vi "Lab4(III).vi"() -> ()   [LabVIEW 2021]
panel:
  out "7":bool
  out "6":bool
  out "3":bool
  out "5":bool
  out "4":bool
  out "2":bool
  out "1":bool
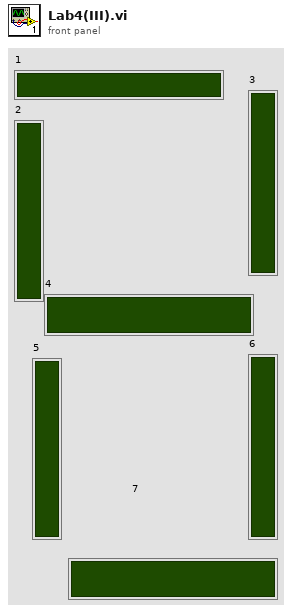
[diagram p1: front panel]
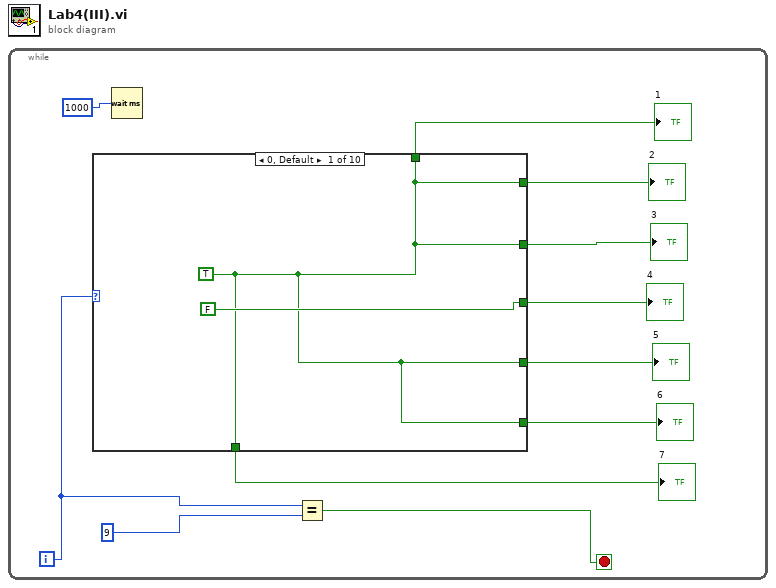
[diagram p0: block diagram]
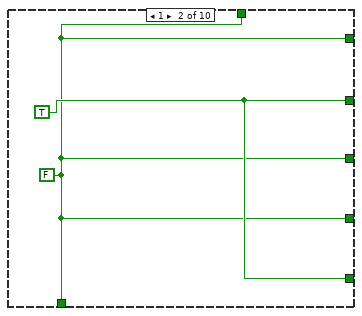
[diagram p2: hidden frame]
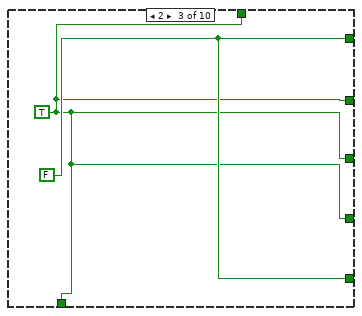
[diagram p3: hidden frame]
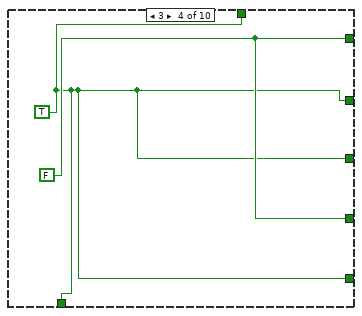
[diagram p4: hidden frame]
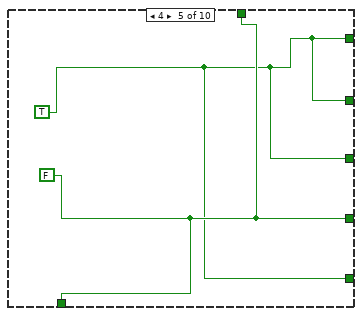
[diagram p5: hidden frame]
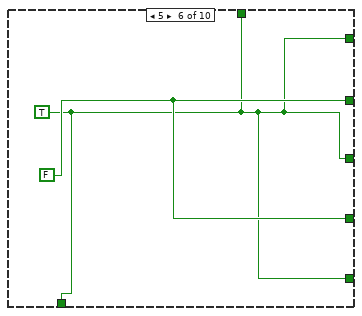
[diagram p6: hidden frame]
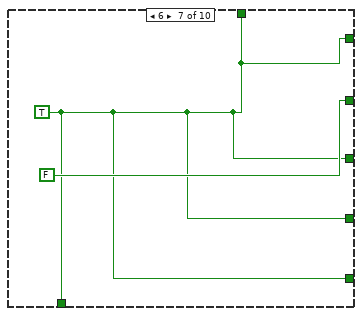
[diagram p7: hidden frame]
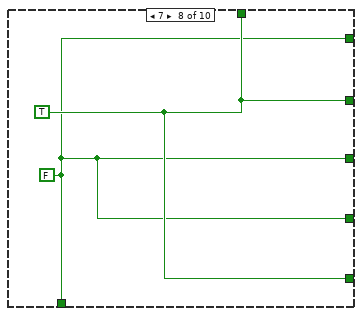
[diagram p8: hidden frame]
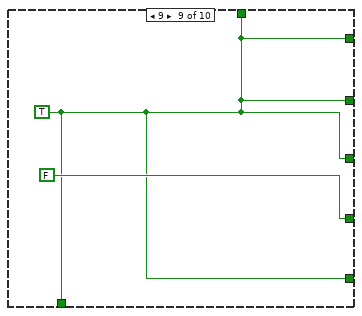
[diagram p9: hidden frame]
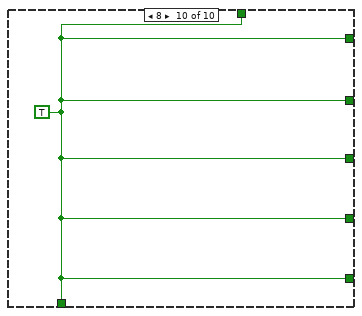
[diagram p10: hidden frame]
diagram:
  n1 = while {
    i -> [w10]
    stop <- w9 stop-if-true
    n2 = case shown="0, Default" w10 {
      tunnel: [w12 w14 w16 w18 w21 w22 w24 w27 w28 w30] -> w8
      tunnel: [w12 w15 w16 w18 w20 w23 FALSE w27 w28 w30] -> w7
      tunnel: [w12 w15 w17 w18 w20 w22 w24 w27 w28 w30] -> w6
      tunnel: [w12 w14 w17 w19 w20 w22 w24 w26 w28 w30] -> w5
      tunnel: [FALSE w14 w16 w18 w20 w22 w24 w26 w28 w30] -> w4
      tunnel: [w12 w14 w16 w19 w21 w23 w24 w26 FALSE w30] -> w3
      tunnel: [w12 w14 w16 w18 w21 w22 w24 w26 w28 w30] -> w2
      frame 0, Default {
        w12 = TRUE
      }
      frame 1 {
        w15 = TRUE
        w14 = FALSE
      }
      frame 2 {
        w16 = TRUE
        w17 = FALSE
      }
      frame 3 {
        w18 = TRUE
        w19 = FALSE
      }
      frame 4 {
        w20 = TRUE
        w21 = FALSE
      }
      frame 5 {
        w22 = TRUE
        w23 = FALSE
      }
      frame 6 {
        w24 = TRUE
      }
      frame 7 {
        w27 = TRUE
        w26 = FALSE
      }
      frame 9 {
        w28 = TRUE
      }
      frame 8 {
        w30 = TRUE
      }
    }
    "1" <- w8
    "2" <- w5
    "4" <- w4
    "5" <- w3
    "3" <- w7
    "6" <- w6
    "7" <- w2
    n3 = Wait (ms)(milliseconds to wait=1000) -> ()  [unwired: 1 out]
    n4 = Equal?(x=w10, y=9) -> (x = y?=w9:bool)
  }
